vi "User Interface.vi"() -> ()   [LabVIEW 2015]
panel:
  in  "D":dbl=0.003
  in  "I":dbl=0.1
  in  "P":dbl=15.0
  out "Lamp Intensity":dbl(slide) scale=0.0..100.0
  out "Temperature":dbl(graph)
  in  "Setpoint":dbl(slide)=25.0 scale=20.0..40.0
  # "Gains"
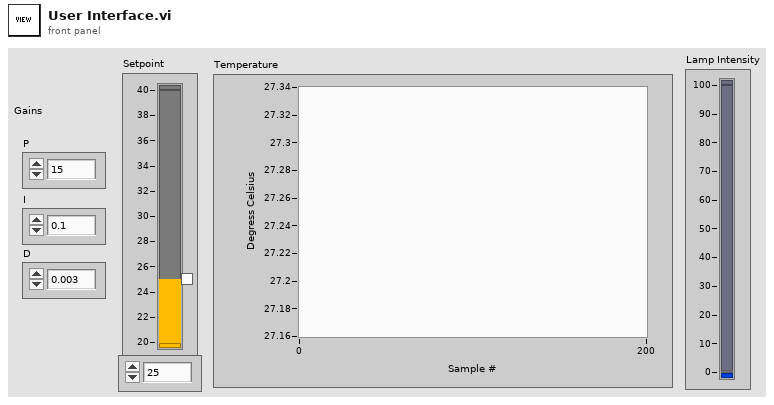
[diagram p1: front panel]
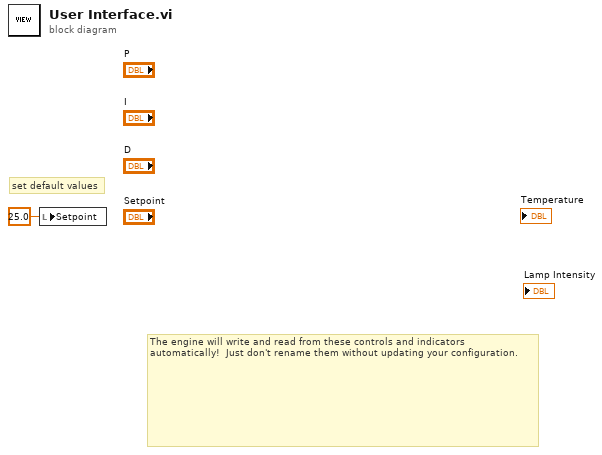
[diagram p0: block diagram]
diagram:
  # "set default values"
  # "The engine will write and read from these controls and indicators automatically!  Just don't rename them without updating your configuration."
  n1 = local write "Setpoint"(25.0 ("Setpoint")) -> ()
